vi "WriteToINIFile.vi"(8 "error in (no error)":errorcluster, 10 "Refnum in":T1, 11 "SiemensDigitalEnergyMeter in":refnum<class "SiemensDigitalEnergyMeter.lvclass">) -> (0 "error out":errorcluster, 3 "SiemensDigitalEnergyMeter out":refnum<class "SiemensDigitalEnergyMeter.lvclass">)   [LabVIEW 2018, in "SensorPlugins.lvlib" / "SiemensDigitalEnergyMeter.lvclass"]
doc: "This VI writes the configuration to the INI file."
uses:
  SiemensDigitalEnergyMeter.lvclass
  <vilib>/Utility/config.llb/Config Data RefNum.ctl
  <vilib>/Utility/config.llb/NI_LVConfig.lvlib
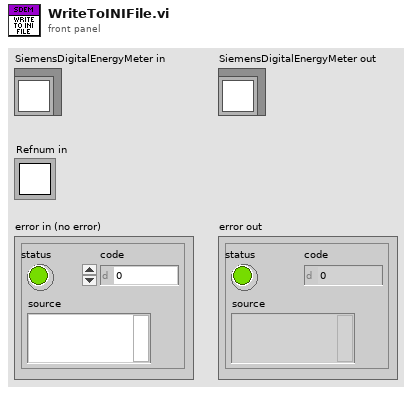
[diagram p1: front panel]
types:
  T1 = typedef "NI_LVConfig.lvlib/Config Data RefNum.ctl" = refnum<k1>
  T2 = typedef "SensorPlugins.lvlib/SiemensDigitalEnergyMeter.lvclass/SiemensDigitalEnergyMeterControls.ctl" = cluster{"Measurement(s)":u16[], "Configuration Commands":string, "Use Measurement Commands Text Box?":bool, "Measurement Commands":string, "Connected?":bool, "Serial Number":string, "IP Address":string, "Port (502)":u16, "Unit ID":u8, "Serial Type":enum16{"RTU", "ASCII"}, "Using TCP?":bool, "VISA Resource Name":string}[]
  T3 = typedef "SensorPlugins.lvlib/SiemensDigitalEnergyMeter.lvclass/MeasurementControls.ctl" = cluster{"Measurement RefreshTime (ms)":u32, "Measurement Name":string}
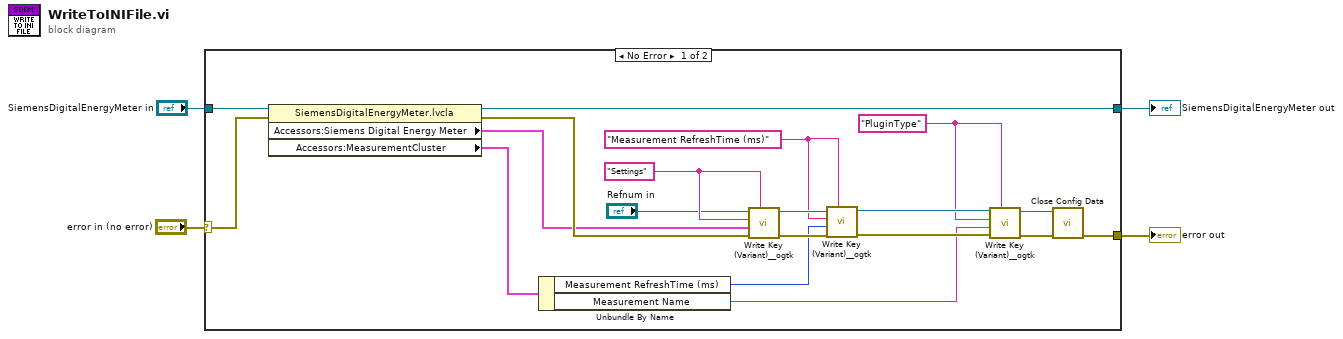
[diagram p0: block diagram]
diagram:
  n1 = case shown="No Error" "error in (no error)" {
    selector: "error in (no error)" -> [w21 w25]
    tunnel: "SiemensDigitalEnergyMeter in" -> [w22 w24]
    tunnel: [w20 w24] -> w2
    tunnel: [w16 w25] -> w1
    frame No Error {
      w5 = "PluginType" ("section (optional)")
      w13 = "Measurement RefreshTime (ms)" ("section (optional)")
      w23 = "Settings" ("section (optional)")
      n2 = property class="SiemensDigitalEnergyMeter.lvcla"(reference=w22, error in=w21) -> (reference out=w20:refnum<class "SiemensDigitalEnergyMeter.lvclass">, error out=w19:errorcluster, "Accessors:Siemens Digital Energy Meter"=w18:T2, "Accessors:MeasurementCluster"=w12:T3)
      n3 = Unbundle By Name(w12) -> ("Measurement RefreshTime (ms)"=w11:u32, "Measurement Name"=w6:string)
      n4 = call <userlib>:"Write Key (Variant)__ogtk.vi"("section"=w23, "error in (no error)"=w19, "key-value"=w18, "key (optional)"=w23, "refnum"="Refnum in") -> ("error out"=w15:errorcluster, "refnum out"=w14:T1)  [unwired: 5 in]
      n5 = call <userlib>:"Write Key (Variant)__ogtk.vi"("section"=w13, "error in (no error)"=w15, "key-value"=w11, "key (optional)"=w13, "refnum"=w14) -> ("error out"=w10:errorcluster, "refnum out"=w9:T1)  [unwired: 5 in]
      n6 = call <userlib>:"Write Key (Variant)__ogtk.vi"("section"=w5, "error in (no error)"=w10, "key-value"=w6, "key (optional)"=w5, "refnum"=w9) -> ("error out"=w8:errorcluster, "refnum out"=w7:T1)  [unwired: 5 in]
      n7 = call <vilib>:"Close Config Data.vi"("error in (no error)"=w8, "refnum"=w7) -> ("error out"=w16:errorcluster)  [unwired: 8 in, 1 out]
    }
    frame Error {
    }
  }
  "error out" <- w1
  "SiemensDigitalEnergyMeter out" <- w2
